vi "DunkFlips.vi"() -> ()   [LabVIEW 2015]
uses:
  <vilib>/rvi/Emulation/niFpgaGetClockAttributes.vi
  <vilib>/rvi/Emulation/niFpgaSctlEmulationGetInTimedLoop.vi
  <vilib>/rvi/Emulation/niFpgaEmulationReportErrorSimple.vi
  <vilib>/rvi/DataTransferAndStorage/Container/Common/niFpgaContainerGetUniqueNameForEmu.vi
  <vilib>/rvi/DataTransferAndStorage/Container/Common/niFpgaContainerSetEmuInfo.vi
  <vilib>/rvi/eio/common/nirviEmuReportErrorAndStop.vi
  <vilib>/rvi/eio/common/nirviEmuTemplateMethod_errors.vi
  <vilib>/rvi/DataTransferAndStorage/Container/Common/niFpgaContainerExecOnDevCompGetState.vi
  <vilib>/rvi/Emulation/niFpgaEmulationIsFPGAContextNoSignature.vi
  <vilib>/rvi/errors/niFpgaSetErrorForExecOnDevCompSimple.vi
  <vilib>/rvi/FIFO/Fifo_Resource/nirvififoEmulationSetSize.vi
  <vilib>/rvi/FIFO/Fifo_Resource/nirviFifoEmulationQueueMgr.vi
  <instcachedir>/0/nirviFifoEmulationQueueMgr_E5CAEC123FF24DC58D834DCA3CDAA9B5.lvgen/nirviFifoEmulationQueueMgr_E5CAEC123FF24DC58D834DCA3CDAA9B5_001.vi
  <vilib>/rvi/FIFO/Fifo_Resource/nirvififoEmulationDetermineInputValidOut.vi
  <vilib>/rvi/FIFO/Fifo_Resource/nirvififoEmulationCreateLock.vi
  <vilib>/rvi/Emulation/niFpgaProcessEmulError.vi
  <vilib>/rvi/FIFO/Fifo_Resource/nirvififoEmulationObtainLock.vi
  <vilib>/rvi/FIFO/Fifo_Resource/nirvififoEmulationReleaseLock.vi
  <vilib>/rvi/occurrence/nirviWaitOnOccurrenceBase.vi
  <vilib>/rvi/errors/nirviReportUnexpectedCaseInternalError.vi
  <vilib>/rvi/errors/nirviReportUnexpectedCaseInternalError (U32).vi
  <vilib>/Utility/error.llb/Clear Errors.vi
  <vilib>/rvi/interface/RandomDataEmulation/niFpgaRandomDataHandleErrors.vi
  <vilib>/rvi/Emulation/niFpgaCriticalErrorInLSC.vi
  <instcachedir>/0/nirviFifoEmulationQueueMgr_E5CAEC123FF24DC58D834DCA3CDAA9B5.lvgen/nirviFifoEmulationQueueMgr_E5CAEC123FF24DC58D834DCA3CDAA9B5_002.vi
  <instcachedir>/0/nirviFifoEmulationQueueMgr_E5CAEC123FF24DC58D834DCA3CDAA9B5.lvgen/nirviFifoEmulationQueueMgr_E5CAEC123FF24DC58D834DCA3CDAA9B5_000.vi
  <vilib>/rvi/LocalResourceManager/LocalResourceManager.xnode
  <vilib>/eio/EIONode/EIONode.xnode
  <vilib>/rvi/DataTransferAndStorage/Container/XNode/niFpgaContainer.xnode
  <vilib>/rvi/FIFO/Fifo_Resource/niFpgaFifoEmulationRefIn.vi
  <vilib>/rvi/interface/RandomDataEmulation/nirviRandomDataFpgaReadWriteTemplate.vi
panel:
  in  "Window Size":fxp<+/-,16,4>
  in  "Threshold":fxp<+/-,16,3>
  out "TDOA 3":i32
  out "TDOA 2":i32
  out "TDOA 1":i32
  out "unsigned value":u16=109
  out "byte value":u16
  out "qfgLO!":i16=109
  in  "Baud Rate":u32=9600
  out "Real Baud Rate":u32=4167
  out "Des BABaus":u32=4167
  out "Actual Sample Period Process (ticks)":u32=80
  in  "Requested Sample Period (ticks)":u32=80
  out "Actual Sample Period Wave (ticks)":u32=80
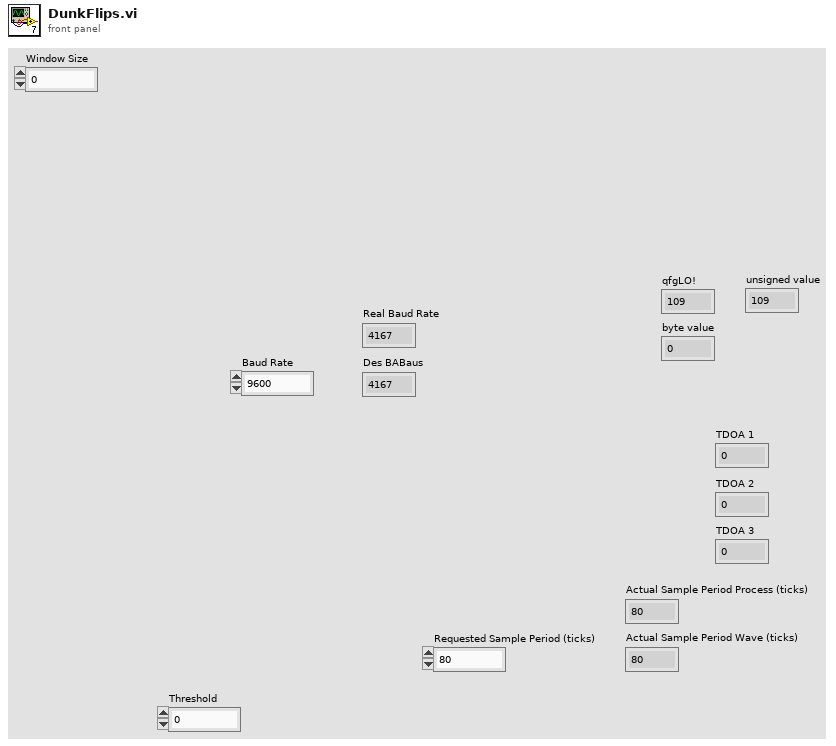
[diagram p1: front panel]
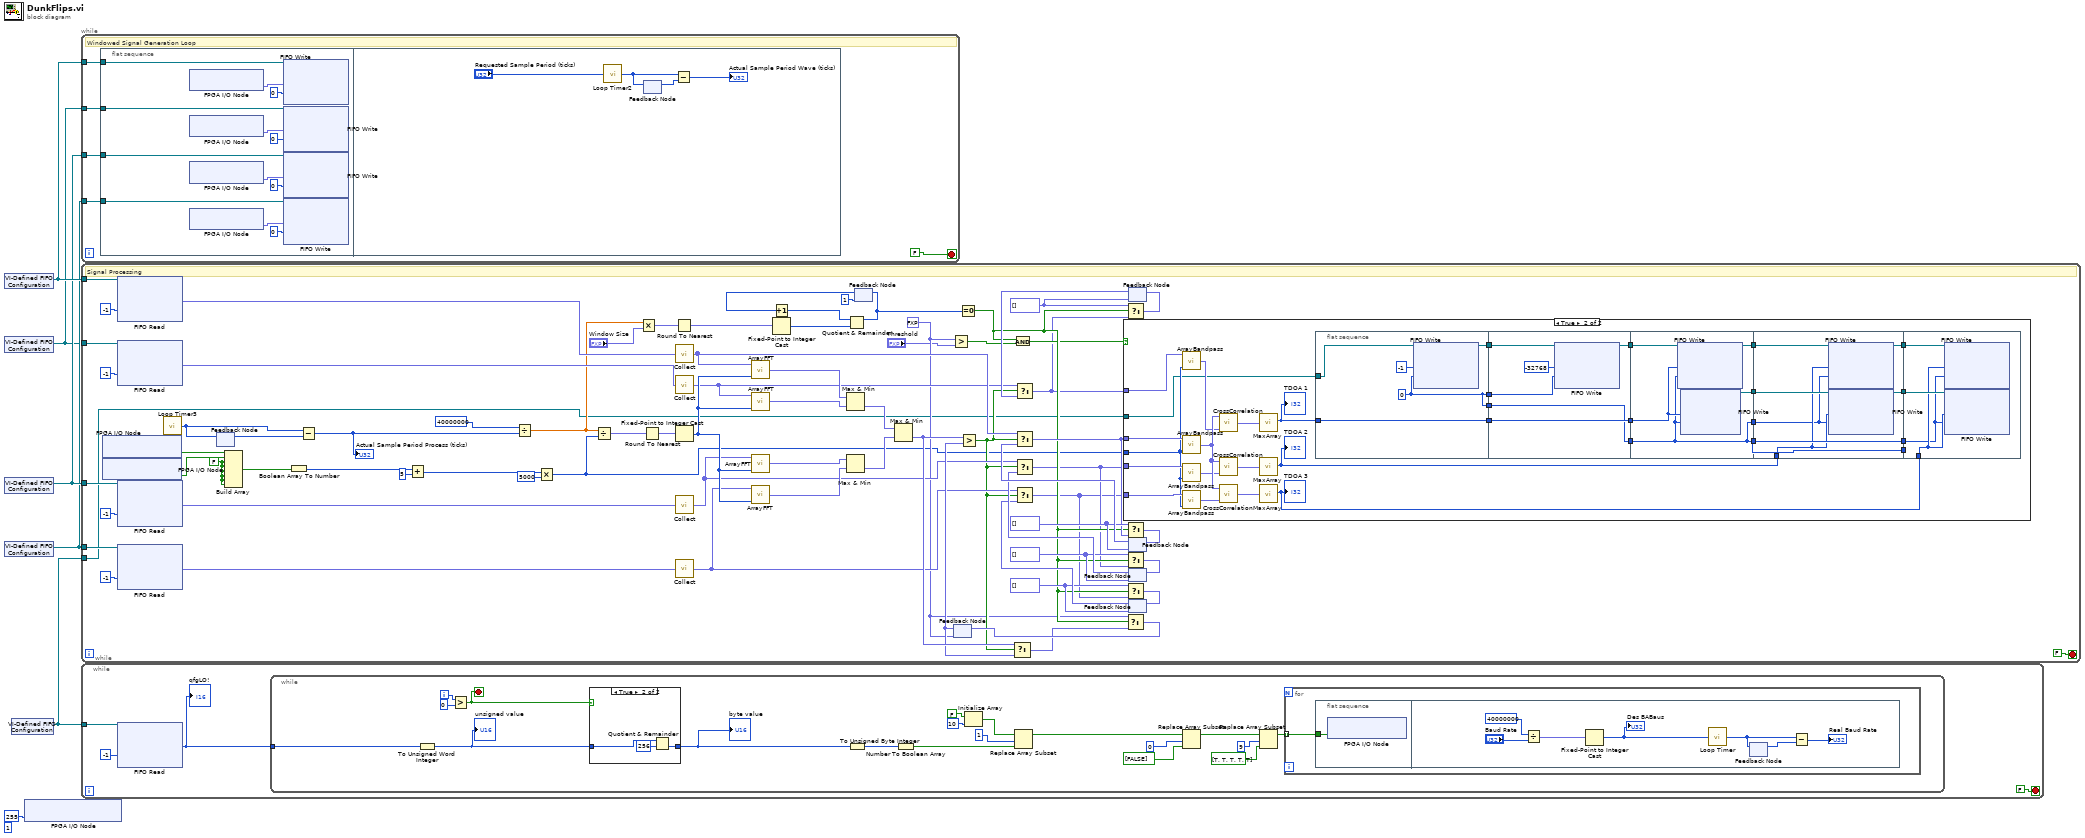
[diagram p0: block diagram]
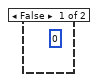
[diagram p3: hidden frame]
diagram:
  (unwired) 1 ("y")
  n1 = xnode "VI-Defined FIFO Configuration"() -> ("FIFO Out"=w6:refnum<k21>)
  n2 = xnode "VI-Defined FIFO Configuration"() -> ("FIFO Out"=w3:refnum<k21>)
  n3 = xnode "VI-Defined FIFO Configuration"() -> ("FIFO Out"=w5:refnum<k21>)
  n4 = xnode "VI-Defined FIFO Configuration"() -> ("FIFO Out"=w4:refnum<k21>)
  n5 = xnode "VI-Defined FIFO Configuration"() -> ("FIFO Out"=w2:refnum<k21>)
  n6 = xnode "FPGA I/O Node"("Connector3/DIOPORT0"=u8 255) -> ()  [unwired: 1 in, 1 out]
  n7 = while {
    tunnel: w6 -> [w11]
    tunnel: w5 -> [w9]
    tunnel: w3 -> [w8]
    tunnel: w4 -> [w7]
    stop <- FALSE stop-if-true
    # "Windowed Signal Generation Loop"
    n8 = flat-sequence {
      tunnel: w11 -> [w18]
      tunnel: w9 -> [w17]
      tunnel: w8 -> [w16]
      tunnel: w7 -> [w19]
      frame #0 {
        n9 = xnode "FPGA I/O Node"() -> ("Connector0/AI0"=w15:fxp<+/-,27,5>)  [unwired: 1 in, 1 out]
        n10 = xnode "FPGA I/O Node"() -> ("Connector0/AI2"=w13:fxp<+/-,27,5>)  [unwired: 1 in, 1 out]
        n11 = xnode "FPGA I/O Node"() -> ("Connector0/AI1"=w12:fxp<+/-,27,5>)  [unwired: 1 in, 1 out]
        n12 = xnode "FPGA I/O Node"() -> ("Connector0/AI3"=w14:fxp<+/-,27,5>)  [unwired: 1 in, 1 out]
        n13 = xnode ("FIFO Write")("Element"=w15, "Timeout"=0, "FIFO In"=w18) -> ()  [unwired: 2 out]
        n14 = xnode ("FIFO Write")("Element"=w13, "Timeout"=0, "FIFO In"=w16) -> ()  [unwired: 2 out]
        n15 = xnode ("FIFO Write")("Element"=w12, "Timeout"=0, "FIFO In"=w17) -> ()  [unwired: 2 out]
        n16 = xnode ("FIFO Write")("Element"=w14, "Timeout"=0, "FIFO In"=w19) -> ()  [unwired: 2 out]
      }
      frame #1 {
        n17 = call "Loop Timer2"("Count(Ticks)"="Requested Sample Period (ticks)") -> ("Tick Count(Ticks)"=w24:u32)
        n18 = feedback #1() -> (w25:u32)  [unwired: 1 in]
        n19 = feedback-in #1(w24) -> ()
        n20 = Subtract(x=w24, y=w25) -> (x-y=→"Actual Sample Period Wave (ticks)":u32)
      }
    }
  }
  n21 = while {
    tunnel: w6 -> [w99]
    tunnel: w5 -> [w100]
    tunnel: w3 -> [w98]
    tunnel: w4 -> [w101]
    tunnel: w2 -> [w30]
    stop <- FALSE stop-if-true
    w43 = fxp<+,16,4>[] []
    w47 = fxp<+,16,4>[] []
    w51 = fxp<+,16,4>[] []
    w54 = fxp<+,16,4>[] []
    w36 = fxp<+/-,16,4> 0.0
    w82 = FALSE
    # "Signal Processing"
    n22 = xnode "FPGA I/O Node"() -> ("Connector2/DIO0"=w85:bool)  [unwired: 1 in, 1 out]
    n23 = xnode "FPGA I/O Node"() -> ("Connector2/DIO1"=w84:bool)  [unwired: 1 in, 1 out]
    n24 = xnode ("FIFO Read")("Timeout"=i16 -1, "FIFO In"=w99) -> ("Element"=w92:fxp<+/-,16,4>)  [unwired: 2 out]
    n25 = xnode ("FIFO Read")("Timeout"=i16 -1, "FIFO In"=w98) -> ("Element"=w91:fxp<+/-,16,4>)  [unwired: 2 out]
    n26 = xnode ("FIFO Read")("Timeout"=i16 -1, "FIFO In"=w100) -> ("Element"=w90:fxp<+/-,16,4>)  [unwired: 2 out]
    n27 = xnode ("FIFO Read")("Timeout"=i16 -1, "FIFO In"=w101) -> ("Element"=w89:fxp<+/-,16,4>)  [unwired: 2 out]
    n28 = call "Loop Timer3"() -> ("Tick Count(Ticks)"=w93:u32)  [unwired: 1 in]
    n29 = feedback #2() -> (w94:u32)  [unwired: 1 in]
    n30 = feedback-in #2(w93) -> ()
    n31 = Build Array(w85, w84, w82, w82, w82, w82, w82, w82) -> (w83:bool[])
    n32 = Boolean Array To Number(Boolean array=w83) -> (number=w81:u8)
    n33 = Subtract(x=w93, y=w94) -> (x-y=w79:u32)
    "Actual Sample Period Process (ticks)" <- w79
    n34 = Add(x=w81, y=i16 5) -> (x+y=w87:i16)
    n35 = Divide(x=40000000, y=w79) -> (x/y=w72:sgl)
    n36 = Multiply(x=w87, y=i16 5000) -> (x*y=w32:u16)
    n37 = Divide(x=w72, y=w32) -> (x/y=w78:fxp<+/-,32,16>)
    n38 = Multiply(x=w72, y="Window Size") -> (x*y=w71:fxp<+/-,32,16>)
    n39 = Round To Nearest(number=w78) -> (nearest integer value=w77:fxp<+/-,17,17>)
    n40 = Round To Nearest(number=w71) -> (nearest integer value=w70:fxp<+/-,17,17>)
    n41 = call "Collect.vi"("Input"=w92) -> ("Output"=w57:fxp<+/-,16,4>[])
    n42 = call "Collect.vi"("Input"=w91) -> ("Output"=w50:fxp<+/-,16,4>[])
    n43 = Fixed-Point to Integer Cast(1:w77) -> (0:w76:i32)
    n44 = call "Collect.vi"("Input"=w90) -> ("Output"=w46:fxp<+/-,16,4>[])
    n45 = call "Collect.vi"("Input"=w89) -> ("Output"=w42:fxp<+/-,16,4>[])
    n46 = call "ArrayFFT.vi"("Period"=w76, "Array"=w57) -> ("Max"=w61:fxp<+,16,4>)  [unwired: 3 in]
    n47 = call "ArrayFFT.vi"("Period"=w76, "Array"=w50) -> ("Max"=w60:fxp<+,16,4>)  [unwired: 3 in]
    n48 = call "ArrayFFT.vi"("Period"=w76, "Array"=w46) -> ("Max"=w59:fxp<+,16,4>)  [unwired: 3 in]
    n49 = call "ArrayFFT.vi"("Period"=w76, "Array"=w42) -> ("Max"=w58:fxp<+,16,4>)  [unwired: 3 in]
    n50 = Fixed-Point to Integer Cast(1:w70) -> (0:w69:i32)
    n51 = Max & Min(x=w61, y=w60) -> (min(x,y)=w65:fxp<+,16,4>)  [unwired: 1 out]
    n52 = Max & Min(x=w59, y=w58) -> (min(x,y)=w64:fxp<+,16,4>)  [unwired: 1 out]
    n53 = feedback #3(u32 1) -> (w74:u32)
    n54 = Increment(x=w74) -> (x+1=w73:u32)
    n55 = Quotient & Remainder(x=w73, y=w69) -> (x-y*floor(x/y)=w67:u32)  [unwired: 1 out]
    n56 = feedback-in #3(w67) -> ()
    n57 = Max & Min(x=w65, y=w64) -> (min(x,y)=w63:fxp<+,16,4>)  [unwired: 1 out]
    n58 = Greater?(x=w36, y="Threshold") -> (0:w37:bool)
    n59 = feedback #4(w36) -> (w62:fxp<+/-,17,5>)
    n60 = Equal To 0?(x=w67) -> (x = 0?=w39:bool)
    n61 = Greater?(x=w63, y=w62) -> (0:w41:bool)
    n62 = Select(t=w63, s=w41, f=w62) -> (s? t:f=w66:fxp<+/-,17,5>)
    n63 = And(x=w39, y=w37) -> (x .and. y?=w38:bool)
    n64 = Select(t=w36, s=w39, f=w66) -> (s? t:f=w68:fxp<+/-,17,5>)
    n65 = feedback-in #4(w68) -> ()
    n66 = feedback #5(w51) -> (w53:fxp<+/-,17,5>[])
    n67 = Select(t=w50, s=w41, f=w53) -> (s? t:f=w35:fxp<+/-,17,5>[])
    n68 = Select(t=w51, s=w39, f=w35) -> (s? t:f=w52:fxp<+/-,17,5>[])
    n69 = feedback-in #5(w52) -> ()
    n70 = feedback #6(w54) -> (w56:fxp<+/-,17,5>[])
    n71 = Select(t=w57, s=w41, f=w56) -> (s? t:f=w40:fxp<+/-,17,5>[])
    n72 = Select(t=w54, s=w39, f=w40) -> (s? t:f=w55:fxp<+/-,17,5>[])
    n73 = feedback-in #6(w55) -> ()
    n74 = feedback #7(w47) -> (w49:fxp<+/-,17,5>[])
    n75 = Select(t=w46, s=w41, f=w49) -> (s? t:f=w34:fxp<+/-,17,5>[])
    n76 = Select(t=w47, s=w39, f=w34) -> (s? t:f=w48:fxp<+/-,17,5>[])
    n77 = feedback-in #7(w48) -> ()
    n78 = feedback #8(w43) -> (w45:fxp<+/-,17,5>[])
    n79 = Select(t=w42, s=w41, f=w45) -> (s? t:f=w33:fxp<+/-,17,5>[])
    n80 = case shown="True" w38 {
      tunnel: w40 -> [_ w133]
      tunnel: w35 -> [_ w132]
      tunnel: w34 -> [_ w131]
      tunnel: w33 -> [_ w130]
      tunnel: w32 -> [_ w129]
      tunnel: w30 -> [_ w106]
      frame False {
        (unwired) i16 0
      }
      frame True {
        n81 = call "ArrayBandpass.vi"("Frequency"=w129, "Input"=w132) -> ("Output"=w127:fxp<+/-,16,4>[])  [unwired: 3 in]
        n82 = call "ArrayBandpass.vi"("Frequency"=w129, "Input"=w133) -> ("Output"=w128:fxp<+/-,16,4>[])  [unwired: 3 in]
        n83 = call "ArrayBandpass.vi"("Frequency"=w129, "Input"=w131) -> ("Output"=w126:fxp<+/-,16,4>[])  [unwired: 3 in]
        n84 = call "ArrayBandpass.vi"("Frequency"=w129, "Input"=w130) -> ("Output"=w125:fxp<+/-,16,4>[])  [unwired: 3 in]
        n85 = call "CrossCorrelation.vi"("Input 2"=w127, "Input 1"=w128) -> ("Output"=w124:fxp<+/-,16,4>[])  [unwired: 3 in]
        n86 = call "CrossCorrelation.vi"("Input 2"=w126, "Input 1"=w128) -> ("Output"=w123:fxp<+/-,16,4>[])  [unwired: 3 in]
        n87 = call "CrossCorrelation.vi"("Input 2"=w125, "Input 1"=w128) -> ("Output"=w122:fxp<+/-,16,4>[])  [unwired: 3 in]
        n88 = call "MaxArray.vi"("Array"=w124) -> ("Max Index"=w105:i32)  [unwired: 3 out]
        "TDOA 1" <- w105
        n89 = call "MaxArray.vi"("Array"=w123) -> ("Max Index"=w104:i32)  [unwired: 3 out]
        "TDOA 2" <- w104
        n90 = call "MaxArray.vi"("Array"=w122) -> ("Max Index"=w103:i32)  [unwired: 3 out]
        "TDOA 3" <- w103
        n91 = flat-sequence {
          tunnel: w105 -> [w138]
          tunnel: [w138] -> w121
          tunnel: [w134] -> w120
          tunnel: w106 -> [w136]
          tunnel: [w135] -> w119
          tunnel: [w134] -> w118
          tunnel: w121 -> [w144]
          tunnel: [w144] -> w117
          tunnel: w120 -> [w143]
          tunnel: [w143] -> w116
          tunnel: w119 -> [w142]
          tunnel: [w141] -> w115
          tunnel: w118 -> [w140]
          tunnel: [w149] -> w114
          tunnel: [w146] -> w113
          tunnel: [w146] -> w112
          tunnel: [w148] -> w111
          tunnel: w117 -> [w147]
          tunnel: w116 -> [w146]
          tunnel: w115 -> [w145]
          tunnel: w114 -> [w156]
          tunnel: [w155] -> w110
          tunnel: w113 -> [w150]
          tunnel: [w154] -> w109
          tunnel: w112 -> [w154]
          tunnel: [w154] -> w108
          tunnel: w104 -> [w151]
          tunnel: w111 -> [w153]
          tunnel: [w152] -> w107
          tunnel: w110 -> [w160]
          tunnel: w109 -> [w157]
          tunnel: w108 -> [_]
          tunnel: w103 -> [w158]
          tunnel: w107 -> [w159]
          frame #0 {
            w134 = i16 0
            n92 = xnode ("FIFO Write")("Element"=i16 -1, "Timeout"=w134, "FIFO In"=w136) -> ("FIFO Out"=w135:refnum<k21>)  [unwired: 1 out]
          }
          frame #1 {
            n93 = xnode ("FIFO Write")("Element"=i16 -32768, "Timeout"=w140, "FIFO In"=w142) -> ("FIFO Out"=w141:refnum<k21>)  [unwired: 1 out]
          }
          frame #2 {
            n94 = xnode ("FIFO Write")("Element"=w147, "Timeout"=w146, "FIFO In"=w145) -> ("FIFO Out"=w148:refnum<k21>)  [unwired: 1 out]
            n95 = xnode ("FIFO Write")("Element"=w147, "Timeout"=w146) -> ("FIFO Out"=w149:refnum<k21>)  [unwired: 1 in, 1 out]
          }
          frame #3 {
            n96 = xnode ("FIFO Write")("Element"=w151, "Timeout"=w150, "FIFO In"=w153) -> ("FIFO Out"=w152:refnum<k21>)  [unwired: 1 out]
            n97 = xnode ("FIFO Write")("Element"=w151, "Timeout"=w150, "FIFO In"=w156) -> ("FIFO Out"=w155:refnum<k21>)  [unwired: 1 out]
          }
          frame #4 {
            n98 = xnode ("FIFO Write")("Element"=w158, "Timeout"=w157, "FIFO In"=w159) -> ()  [unwired: 2 out]
            n99 = xnode ("FIFO Write")("Element"=w158, "Timeout"=w157, "FIFO In"=w160) -> ()  [unwired: 2 out]
          }
        }
      }
    }
    n100 = Select(t=w43, s=w39, f=w33) -> (s? t:f=w44:fxp<+/-,17,5>[])
    n101 = feedback-in #8(w44) -> ()
  }
  n102 = while {
    tunnel: w2 -> [w164]
    stop <- FALSE stop-if-true
    n103 = xnode ("FIFO Read")("Timeout"=i16 -1, "FIFO In"=w164) -> ("Element"=w161:i16)  [unwired: 2 out]
    "qfgLO!" <- w161
    n104 = while {
      tunnel: w161 -> [w170]
      i -> [w168]
      stop <- w165 stop-if-true
      n105 = To Unsigned Word Integer(number=w170) -> (unsigned 16bit integer=w169:u16)
      "unsigned value" <- w169
      n106 = Greater?(x=w168, y=i16 0) -> (0:w165:bool)
      n107 = case shown="True" w165 {
        tunnel: [w184 w185] -> w167
        tunnel: w169 -> [w184 w187]
        frame False {
        }
        frame True {
          n108 = Quotient & Remainder(x=w187, y=u16 256) -> (floor(x/y)=w185:u16)  [unwired: 1 out]
        }
      }
      "byte value" <- w167
      n109 = To Unsigned Byte Integer(number=w167) -> (unsigned 8bit integer=w166:u8)
      n110 = Number To Boolean Array(number=w166) -> (Boolean array=w175:bool[])
      n111 = Initialize Array(FALSE, i16 10) -> (w173:bool[])
      n112 = Replace Array Subset(array=w173, new element=w175, index=1) -> (w176:bool[])
      n113 = Replace Array Subset(array=w176, new element=bool[] [FALSE], index=0) -> (w181:bool[])
      n114 = Replace Array Subset(array=w181, new element=bool[] [TRUE, TRUE, TRUE, TRUE, TRUE], index=9) -> (w182:bool[])
      n115 = for {
        tunnel: w182 -> [w188] mode=indexing
        n116 = flat-sequence {
          tunnel: w188 -> [w189]
          frame #0 {
            n117 = xnode "FPGA I/O Node"("Connector1/DIO0"=w189) -> ()  [unwired: 1 in, 1 out]
          }
          frame #1 {
            n118 = Divide(x=40000000, y="Baud Rate") -> (x/y=w191:fxp<+/-,16,16>)
            n119 = Fixed-Point to Integer Cast(1:w191) -> (0:w190:i16)
            "Des BABaus" <- w190
            n120 = call "Loop Timer"("Count(Ticks)"=w190) -> ("Tick Count(Ticks)"=w194:u32)
            n121 = feedback #9() -> (w195:u32)  [unwired: 1 in]
            n122 = feedback-in #9(w194) -> ()
            n123 = Subtract(x=w194, y=w195) -> (x-y=→"Real Baud Rate":u32)
          }
        }
      }
    }
  }
